vi "Send 90 Degree Pulse Command.vi"(6 "Pulse Sequence Type":T1, 8 "error in (no error)":errorcluster, 11 "class objects in":T2) -> (0 "error out":errorcluster, 2 "CMD STR Array":string[](array[string]), 3 "class objects out":T2)   [LabVIEW 2011]
uses:
  Controls/Class Objects2.ctl
  Modules/File/Configuration/Configuration.lvclass
  Modules/Hardware/Power Supply/Power Supply.lvclass
  Modules/Hardware/NMR/NMR.lvclass
  Modules/File/TDMS/TDMS.lvclass
  Controls/NMR Pulse Sequence Type.ctl
  Controls/TDMS File Handling.ctl
  Functional Globals/Pulse Parameters.ctl
  Controls/User Interface Action2.ctl
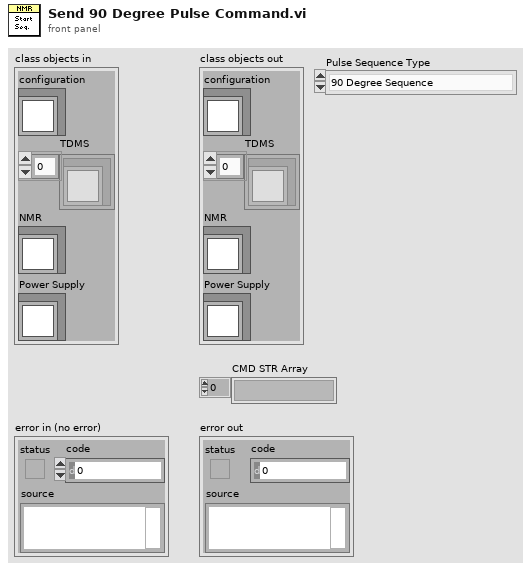
[diagram p1: front panel]
types:
  T1 = typedef "NMR Pulse Sequence Type.ctl" = enum16{"90 Degree Sequence", "CMPG Pulse Sequence", "T1 Pulse Sequence"}
  T2 = typedef "Class Objects2.ctl" = cluster{"configuration":refnum<class "Configuration.lvclass">, "TDMS":refnum<class "TDMS.lvclass">[], "Power Supply":refnum<class "Power Supply.lvclass">, "NMR":refnum<class "NMR.lvclass">}
  T3 = typedef "TDMS File Handling.ctl" = enum16{"Add TDMS File", "Get Active TDMS File", "Set Active TDMS File", "Set Active TDMS File Index"}
  T4 = typedef "Pulse Parameters.ctl" = enum16{"Initialize", "Set T1 Pulse Settings", "Set 90 Degree Pulse Settings", "Set CPMG Pulse Settings", "Get T1 Pulse Settings", "Get 90 Degree Pulse Settings", "Get T1 Settings", "Get CPMG Settings", "Get 90 Degree Settings", "Get CPMG Pulse Settings"}
  T5 = typedef "User Interface Action2.ctl" = enum16{"Initialize", "Update Real Channel", "Update Imag Channel", "Update Real FFT Channel", "Update Imag FFT Channel", "Pulse Sequence", "Visibility Front Panel Controls", "Report Custom Errors", "Visibility Pulse Parameters", "Update Pulse Timings", "Update Status Bar", "Stop"}
  T6 = typedef "Full_90 Degree Pulse Settings.ctl" = cluster{"Delay Settings":T7, "Preliminary Settings":T8, "Pulse Settings":T9, "Acquisition Settings":T10}
  T7 = typedef "90D_Delay Settings.ctl" = cluster{"Delay d1":dbl, "Delay d2":dbl, "d1 Unit":u8, "d2 Unit":u8}
  T8 = typedef "90D_Preliminary Settings.ctl" = cluster{"Nº of Scans (ns)":u16, "Pulse Frequency":dbl}
  T9 = typedef "90D_Pulse Settings.ctl" = cluster{"Duration Signal P1":dbl, "Power Level":u16, "Phase":u16, "P1 Units":u8}
  T10 = typedef "Acquisition Settings.ctl" = cluster{"Number Samples":u16, "Time Between Points":dbl, "Unit":u8}
  T11 = cluster{"D1 Real Time":ext, "D2 Real Time":ext, "P1 Real Time":ext, "AQS Real Time":ext}
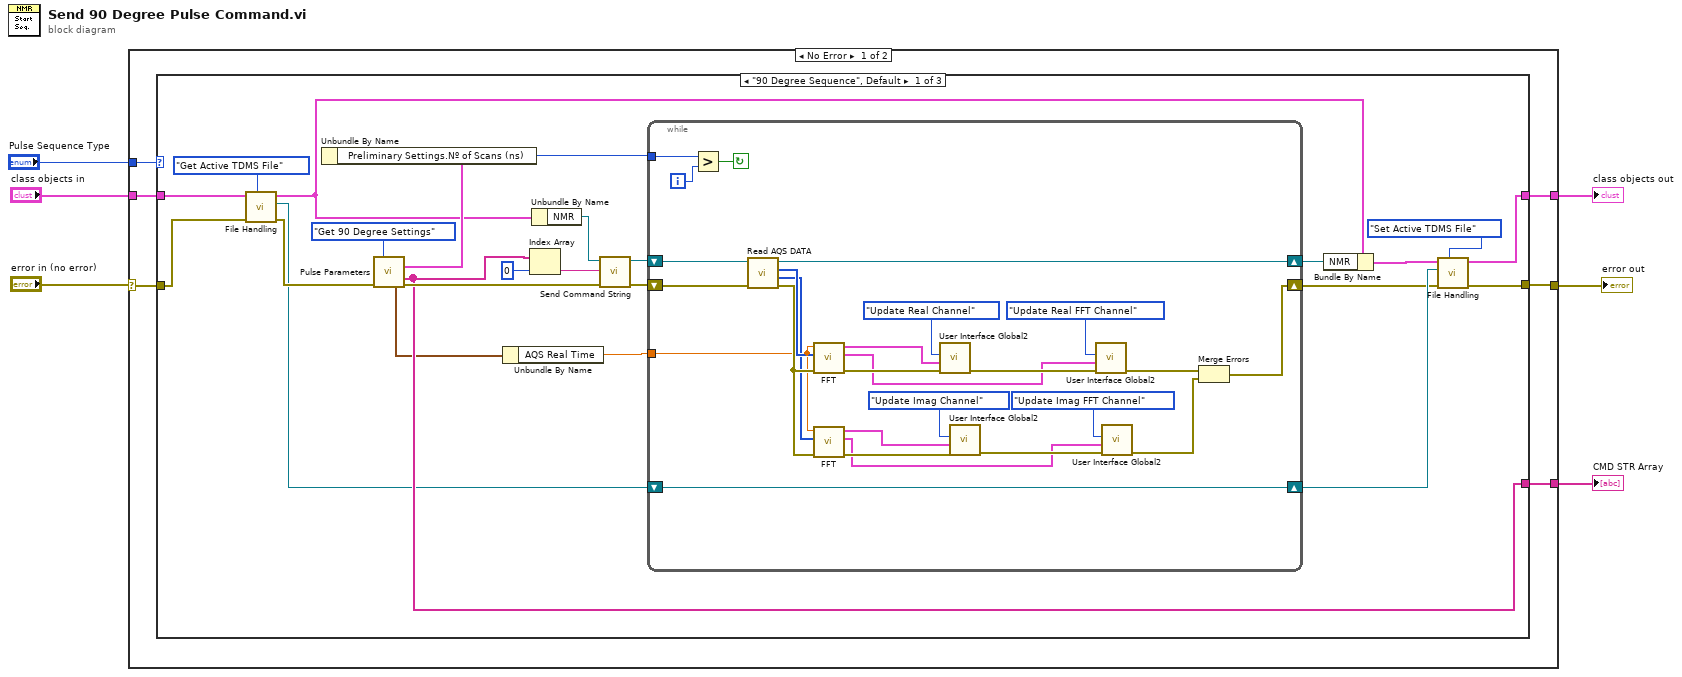
[diagram p0: block diagram]
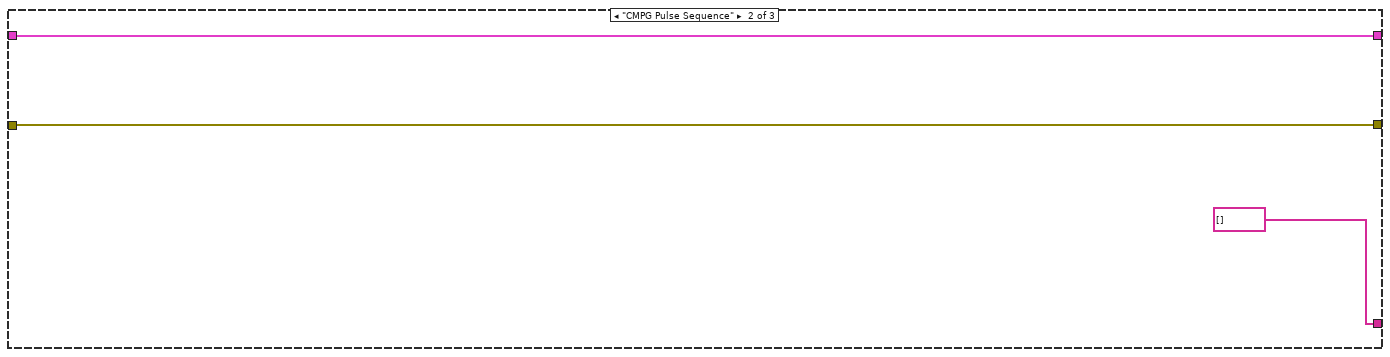
[diagram p2: hidden frame]
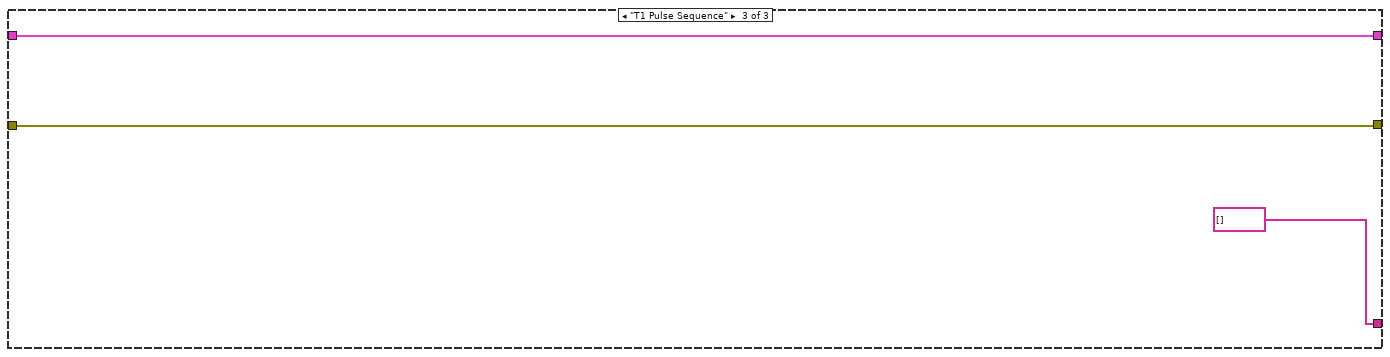
[diagram p3: hidden frame]
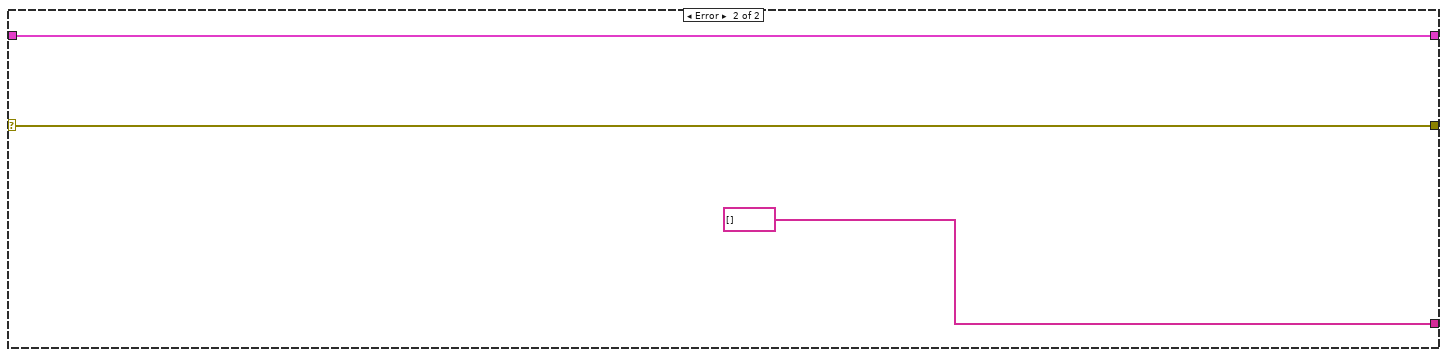
[diagram p4: hidden frame]
diagram:
  n1 = case shown="No Error" "error in (no error)" {
    selector: "error in (no error)" -> [w9 w71]
    tunnel: [w12 string[] [] ("CMD STR Array")] -> w6
    tunnel: [w11 w72] -> w5
    tunnel: "class objects in" -> [w10 w72]
    tunnel: [w8 w71] -> w3
    tunnel: "Pulse Sequence Type" -> [w7 _]
    frame No Error {
      n2 = case shown="\"90 Degree Sequence\", Default" w7 {
        tunnel: [w31 string[] [] ("CMD STR Array") string[] [] ("CMD STR Array")] -> w12
        tunnel: [w13 w66 w69] -> w11
        tunnel: w10 -> [w24 w66 w69]
        tunnel: w9 -> [w21 w65 w68]
        tunnel: [w15 w65 w68] -> w8
        frame "90 Degree Sequence", Default {
          n3 = call "File Handling.vi"("TDMS File Handling"=TDMS_File_Handling."Get Active TDMS File", "error in"=w21, "objects IN"=w24) -> ("error out"=w20:errorcluster, "TDMS File"=w19:refnum<class "TDMS.lvclass">, "objects OUT"=w23:T2)  [unwired: 6 in]
          n4 = call "Pulse Parameters.vi"("action"=Pulse_Parameters."Get 90 Degree Settings", "error in"=w20) -> ("90 Degree Pulse Sequence OUT"=w36:T6, "CMD STR Array"=w31:string[], "Set Time 90 Degree Pulse"=w26:T11, "error out"=w32:errorcluster)  [unwired: 8 in, 2 out]
          n5 = Unbundle By Name(w36) -> ("Preliminary Settings.Nº of Scans (ns)"=w35:u16)
          n6 = Unbundle By Name(w26) -> ("AQS Real Time"=w25:ext)
          n7 = Index Array(array=w31, index=0) -> (element=w30:string)
          n8 = Unbundle By Name(w23) -> ("NMR"=w33:refnum<class "NMR.lvclass">)
          n9 = call-dynamic "Send Command String.vi"("error in (no error)"=w32, "Command String"=w30, "NMR in"=w33) -> ("error out"=w28:errorcluster, "NMR out"=w29:refnum<class "NMR.lvclass">)  [unwired: 7 in]
          n10 = while {
            tunnel: w35 -> [w45]
            shift-right: [w42] -> w27
            shift-left: w29 -> [w43]
            shift-right: [w41] -> w16
            shift-left: w28 -> [w40]
            tunnel: w25 -> [w39]
            shift-right: [w38] -> w17
            shift-left: w19 -> [w38]
            i -> [w46]
            stop <- w44 continue-if-true
            n11 = Greater?(x=w45, y=w46) -> (0:w44:bool)
            n12 = call-dynamic "Read AQS DATA.vi"("error in (no error)"=w40, "NMR in"=w43) -> ("error out"=w63:errorcluster, "Imag Data"=w61:i32[], "Real Data"=w62:i32[], "NMR out"=w42:refnum<class "NMR.lvclass">)  [unwired: 6 in]
            n13 = call "FFT.vi"("error in (no error)"=w63, "Input Array"=w62, "Delay Sample"=w39) -> ("error out"=w59:errorcluster, "Time Graph"=w55:cluster{"magnitude":dbl[], dbl[]}, "FFT Graph"=w60:cluster{"magnitude":dbl[], dbl[]})  [unwired: 6 in]
            n14 = call "FFT.vi"("error in (no error)"=w63, "Input Array"=w61, "Delay Sample"=w39) -> ("error out"=w51:errorcluster, "Time Graph"=w49:cluster{"magnitude":dbl[], dbl[]}, "FFT Graph"=w50:cluster{"magnitude":dbl[], dbl[]})  [unwired: 6 in]
            n15 = call "User Interface Global2.vi"("error in"=w59, "data1"=w60, "action"=User_Interface_Action2."Update Real Channel") -> ("error out"=w56:errorcluster)  [unwired: 8 in]
            n16 = call "User Interface Global2.vi"("error in"=w51, "data1"=w50, "action"=User_Interface_Action2."Update Imag Channel") -> ("error out"=w52:errorcluster)  [unwired: 8 in]
            n17 = call "User Interface Global2.vi"("error in"=w56, "data1"=w55, "action"=User_Interface_Action2."Update Real FFT Channel") -> ("error out"=w48:errorcluster)  [unwired: 8 in]
            n18 = call "User Interface Global2.vi"("error in"=w52, "data1"=w49, "action"=User_Interface_Action2."Update Imag FFT Channel") -> ("error out"=w47:errorcluster)  [unwired: 8 in]
            n19 = Merge Errors(w48, w47) -> (w41:errorcluster)
          }
          n20 = Bundle By Name(cluster=w23, "NMR"=w27) -> (w14:T2)
          n21 = call "File Handling.vi"("TDMS File Handling"=TDMS_File_Handling."Set Active TDMS File", "error in"=w16, "TDMS File"=w17, "objects IN"=w14) -> ("error out"=w15:errorcluster, "objects OUT"=w13:T2)  [unwired: 5 in, 1 out]
        }
        frame "CMPG Pulse Sequence" {
        }
        frame "T1 Pulse Sequence" {
        }
      }
    }
    frame Error {
    }
  }
  "CMD STR Array" <- w6
  "class objects out" <- w5
  "error out" <- w3
